vi "MethodCreationList.vi"() -> ()   [LabVIEW 2020]
uses:
  <vilib>/Utility/miscctls.llb/LVRowAndColumnUnsignedTypeDef.ctl
  93525925-75d2-4d3a-a9f9-1ccb6577911a.vi
  3f7d870a-561c-45f8-97df-b7155e0f9951.vi
panel:
  in  "_":string[][](table) caption="3 methods selected"
  out "Over":i32(listbox) caption="Over\nride?"
  out "Listbox":i32(listbox)
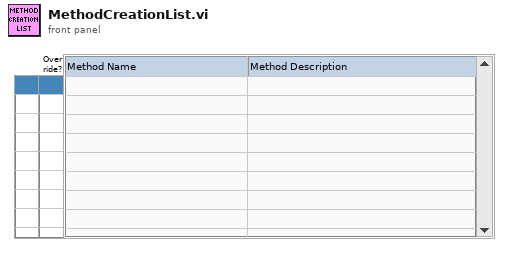
[diagram p1: front panel]
types:
  T1 = typedef "LVRowAndColumnUnsignedTypeDef.ctl" = cluster{"Row":u32, "Column":u32}
  T2 = typedef "LVPoint32TypeDef.ctl" = cluster{"Horizontal":i32, "Vertical":i32}
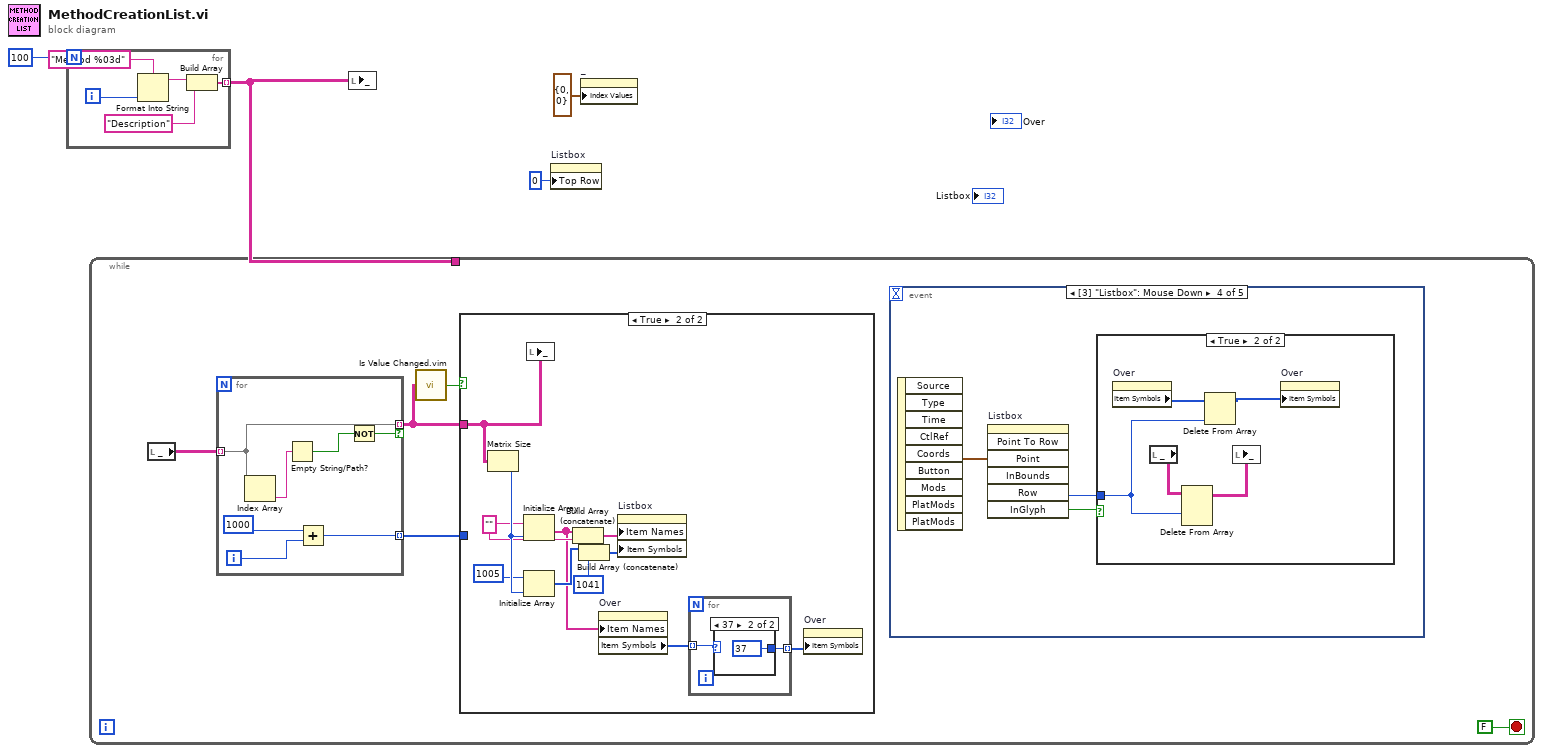
[diagram p0: block diagram]
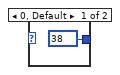
[diagram p3: hidden frame]
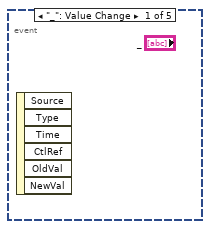
[diagram p4: hidden frame]
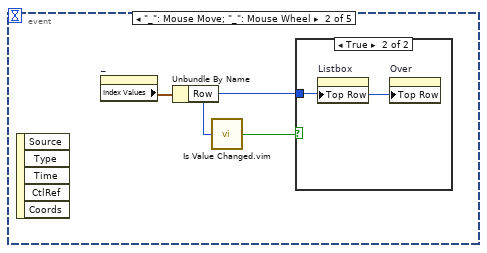
[diagram p5: hidden frame]
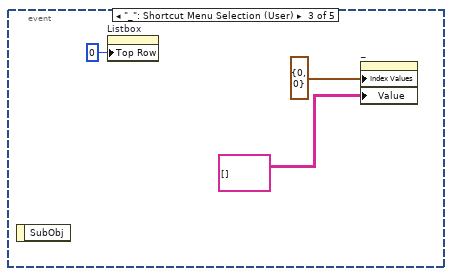
[diagram p7: hidden frame]
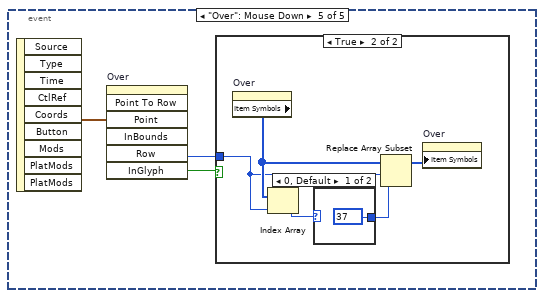
[diagram p9: hidden frame]
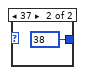
[diagram p11: hidden frame]
diagram:
  n1 = for {
    N: 100 -> [_]
    tunnel: [w5] -> w3 mode=indexing
    i -> [w8]
    n2 = Format Into String(format string="Method %03d", w8) -> (resulting string=w7:string)  [unwired: 2 in, 1 out]
    n3 = Build Array(w7, "Description" ("format string")) -> (w5:string[])
  }
  n4 = while {
    tunnel: w3 -> [_]
    stop <- FALSE stop-if-true
    n5 = local read "_"() -> (w13:string[][])
    n6 = for {
      tunnel: w13 -> [w34] mode=indexing
      tunnel: [w34] -> w12 mode=indexing if=w36
      tunnel: [w30] -> w10 mode=indexing
      i -> [w31]
      n7 = Index Array(array=w34) -> (element=w35:string)  [unwired: 1 in]
      n8 = Empty String/Path?(string/path=w35) -> (empty?=w33:bool)
      n9 = Add(x=1000 ("y"), y=w31) -> (x+y=w30:i32)
      n10 = Not(x=w33) -> (.not. x?=w36:bool)
    }
    n11 = call "Is Value Changed.vim"("value"=w12) -> ("changed or first call?"=w11:bool)
    n12 = case shown="True" w11 {
      tunnel: w12 -> [_ w25]
      tunnel: w10 -> [_ _]
      frame False {
      }
      frame True {
        w19 = ""
        n13 = Matrix Size(0:w25) -> (1:w24:i32)  [unwired: 1 out]
        n14 = Initialize Array(w19, w24) -> (w17:string[])
        n15 = Initialize Array(1005 ("y"), w24) -> (w23:i32[])
        n16 = local write "_"(w25) -> ()
        n17 = Build Array (concatenate)(w17, w19) -> (w21:string[])
        n18 = Build Array (concatenate)(w23, 1041 ("y")) -> (w20:i32[])
        n19 = property on="Over" class="LstBox (strict)"("Item Names"=w17) -> ("Item Symbols"=w16:i32[])  [unwired: 2 in, 2 out]
        n20 = property on="Listbox" class="LstBox (strict)"("Item Names"=w21, "Item Symbols"=w20) -> ()  [unwired: 2 in, 2 out]
        n21 = for {
          tunnel: w16 -> [w27] mode=indexing
          tunnel: [w26] -> w15 mode=indexing
          n22 = case shown="37" w27 {
            tunnel: [38 37] -> w26
            frame 0, Default {
            }
            frame 37 {
            }
          }
        }
        n23 = property on="Over" class="LstBox (strict)"("Item Symbols"=w15) -> ()  [unwired: 2 in, 2 out]
      }
    }
    n24 = event shown="[3] \"Listbox\": Mouse Down" {
      selector: _ -> [_ _ _ _ _]
      dyn-events: _ -> [_ _ _ _ _]
      timeout: _ -> [_ _ _ _ _]
      event "_": Value Change {
        n25 = event-data() -> ()  [unwired: 1 in, 6 out]
      }
      event "_": Mouse Move; "_": Mouse Wheel {
        n26 = event-data() -> ()  [unwired: 1 in, 5 out]
        n27 = property on="_" class="Tbl (strict)"() -> ("Index Values"=w39:T1)  [unwired: 2 in, 2 out]
        n28 = Unbundle By Name(w39) -> ("Row"=w38:u32)
        n29 = call "Is Value Changed.vim"("value"=w38) -> ("changed or first call?"=w37:bool)
        n30 = case shown="True" w37 {
          tunnel: w38 -> [_ w40]
          frame False {
          }
          frame True {
            n31 = property on="Listbox" class="LstBox (strict)"("Top Row"=w40) -> ()  [unwired: 2 in, 2 out]
            n32 = property on="Over" class="LstBox (strict)"("Top Row"=w40) -> ()  [unwired: 2 in, 2 out]
          }
        }
      }
      event "_": Shortcut Menu Selection (User) {
        n33 = event-data() -> ()  [unwired: 1 in, 1 out]
        n34 = property on="Listbox" class="LstBox (strict)"("Top Row"=0) -> ()  [unwired: 2 in, 2 out]
        n35 = property on="_" class="Tbl (strict)"("Index Values"=T1 {"Row"=0, "Column"=0}, "Value"=string[][] [] ("Methods")) -> ()  [unwired: 2 in, 2 out]
      }
      event "Listbox": Mouse Down {
        n36 = event-data() -> ("Coords"=w46:T2)  [unwired: 1 in, 8 out]
        n37 = invoke on="Listbox" class="LstBox (strict)" method="Point To Row"("Point"=w46) -> ("Row"=w44:i32, "InGlyph"=w45:bool)  [unwired: 6 in, 5 out]
        n38 = case shown="True" w45 {
          tunnel: w44 -> [_ w48]
          frame False {
          }
          frame True {
            n39 = property on="Over" class="LstBox (strict)"() -> ("Item Symbols"=w49:i32[])  [unwired: 2 in, 2 out]
            n40 = local read "_"() -> (w51:string[][])
            n41 = Delete From Array(array=w51, index (row)=w48) -> (array with subset deleted=w50:string[][])  [unwired: 2 in, 1 out]
            n42 = Delete From Array(array=w49, index=w48) -> (array with subset deleted=w47:i32[])  [unwired: 1 in, 1 out]
            n43 = local write "_"(w50) -> ()
            n44 = property on="Over" class="LstBox (strict)"("Item Symbols"=w47) -> ()  [unwired: 2 in, 2 out]
          }
        }
      }
      event "Over": Mouse Down {
        n45 = event-data() -> ("Coords"=w54:T2)  [unwired: 1 in, 8 out]
        n46 = invoke on="Over" class="LstBox (strict)" method="Point To Row"("Point"=w54) -> ("Row"=w52:i32, "InGlyph"=w53:bool)  [unwired: 6 in, 5 out]
        n47 = case shown="True" w53 {
          tunnel: w52 -> [_ w57]
          frame False {
          }
          frame True {
            n48 = property on="Over" class="LstBox (strict)"() -> ("Item Symbols"=w58:i32[])  [unwired: 2 in, 2 out]
            n49 = Index Array(array=w58, index=w57) -> (element=w56:i32)
            n50 = case shown="0, Default" w56 {
              tunnel: [37 38] -> w55
              frame 0, Default {
              }
              frame 37 {
              }
            }
            n51 = Replace Array Subset(array=w58, new element=w55, index=w57) -> (w59:i32[])
            n52 = property on="Over" class="LstBox (strict)"("Item Symbols"=w59) -> ()  [unwired: 2 in, 2 out]
          }
        }
      }
    }
  }
  n53 = local write "_"(w3) -> ()
  n54 = property on="Listbox" class="LstBox (strict)"("Top Row"=0) -> ()  [unwired: 2 in, 2 out]
  n55 = property on="_" class="Tbl (strict)"("Index Values"=T1 {"Row"=0, "Column"=0}) -> ()  [unwired: 2 in, 2 out]
